vi "PID Angle.vi"(10 "Enable?":bool, 11 "Angle to Goal":dbl) -> (3 "Frame Velocity":dbl[](array[numeric]))   [LabVIEW 2016]
uses:
  <vilib>/addons/control/pid/pid.llb/PID (DBL).vi
  <vilib>/addons/control/pid/NI_PID_pid.lvlib
panel:
  out "PID Value":dbl
  in  "PID gains":T1={"proportional gain (Kc)"=0.7, "integral time (Ti, min)"=0.0, "derivative time (Td, min)"=0.0}
  out "Goal Arrive?":bool
  in  "Direction to Goal":T2
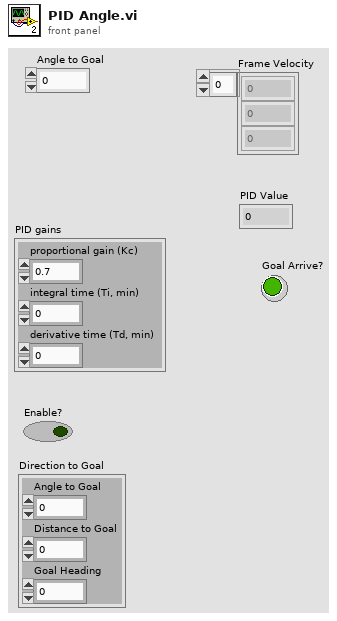
[diagram p1: front panel]
types:
  T1 = cluster{"proportional gain (Kc)":dbl, "integral time (Ti, min)":dbl, "derivative time (Td, min)":dbl}
  T2 = cluster{"Angle to Goal":dbl, "Distance to Goal":sgl, "Goal Heading":sgl}
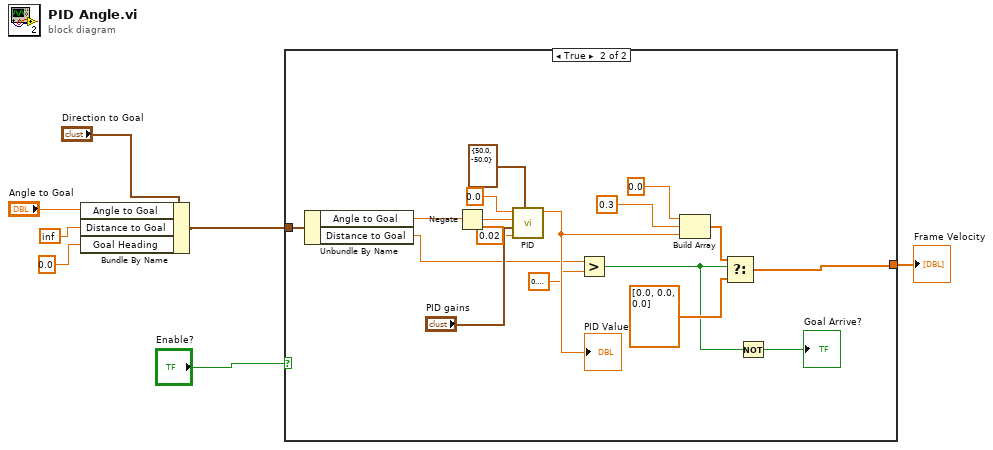
[diagram p0: block diagram]
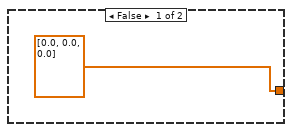
[diagram p2: hidden frame]
diagram:
  n1 = Bundle By Name(cluster="Direction to Goal", "Angle to Goal"="Angle to Goal", "Distance to Goal"=inf, "Goal Heading"=sgl 0.0) -> (w2:T2)
  n2 = case shown="True" "Enable?" {
    tunnel: w2 -> [_ w19]
    tunnel: [dbl[] [0.0, 0.0, 0.0] ("Frame Velocity") w9] -> w1
    frame False {
    }
    frame True {
      n3 = Unbundle By Name(w19) -> ("Angle to Goal"=w20:dbl, "Distance to Goal"=w17:sgl)
      n4 = Negate(x=w20) -> (-x=w21:dbl)
      n5 = call-poly <vilib>:"PID.vi"("output range"=cluster{"output high":dbl, "output low":dbl} {"output high"=50.0, "output low"=-50.0}, "dt (s)"=0.02, "PID gains"="PID gains", "process variable"=w21, "setpoint"=0.0) -> ("output"=w24:dbl)  [unwired: 5 in, 1 out]
      "PID Value" <- w24
      n6 = Greater?(x=w17, y=sgl 0.3) -> (0:w12:bool)
      n7 = Build Array(0.0 ("element"), 0.3 ("element"), w24) -> (w14:dbl[])
      n8 = Select(t=w14, s=w12, f=dbl[] [0.0, 0.0, 0.0]) -> (s? t:f=w9:dbl[])
      n9 = Not(x=w12) -> (.not. x?=→"Goal Arrive?":bool)
    }
  }
  "Frame Velocity" <- w1
